vi "Write Return Address and Payload.vi"(7 "Reply Message":refnum<class "Message.lvclass">, 9 "Return Priority (Normal)":T1=enum."Normal", 10 "Return Address":refnum<class "Message Enqueuer.lvclass">, 11 "Dialog Return Msg in":refnum<class "Dialog Return Msg.lvclass">) -> (3 "Dialog Return Msg out":refnum<class "Dialog Return Msg.lvclass">)   [LabVIEW 2020, in "IDialogBox.lvlib" / "Dialog Return Msg.lvclass"]
doc: "<License>\nCopyright © 2017 Composed Systems, LLC | All rights reserved\nwww.composed.io\n\nAuthor: Ethan Stern <ethan.stern@composed.io>\n\nThis software is provided \"AS IS\" WITHOUT WARRANTIES, either express or implied, AND IS FOR EDUCATIONAL PURPOSES ONLY.\n</License>"
uses:
  Dialog Return Msg.lvclass
  <vilib>/ActorFramework/Message/Message.lvclass
  <vilib>/ActorFramework/Message Enqueuer/Message Enqueuer.lvclass
  <vilib>/ActorFramework/Message Enqueuer/Message Priority.ctl
  Dialog Return Msg.lvclass/Dialog Return Msg.ctl
panel:
  # "This input is here in case\nany future Actors want to\noverride the Dialog Return Msg.\nIf unwired, this method just\ninstantiates the basic message\ntype, which is good enough\nfor most reply scenarios."
  # "此输入用于以防万一\n任何未来的演员都想\n覆盖对话框返回消息。\n如果未布线，此方法只是\n实例化基本消息\n类型，这已经足够好了\n对于大多数回复场景。"
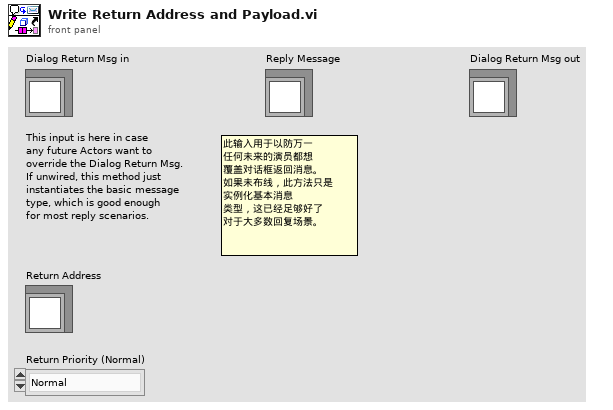
[diagram p1: front panel]
types:
  T1 = typedef "Actor Framework.lvlib/Message Enqueuer.lvclass/Message Priority.ctl" = enum16{"Low", "Normal", "High"}
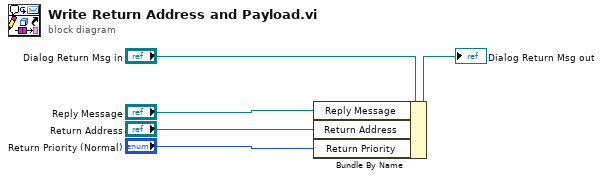
[diagram p0: block diagram]
diagram:
  n1 = Bundle By Name(cluster="Dialog Return Msg in", "Reply Message"="Reply Message", "Return Address"="Return Address", "Return Priority"="Return Priority (Normal)") -> (→"Dialog Return Msg out":refnum<class "Dialog Return Msg.lvclass">)
